vi "test_read-nmea-data2.vi"() -> ()   [LabVIEW 2019] (continued)
$GNGLL,3723.59722,N,12656.90157,E,060937.00,A,A*7E\n\t\n15:09:35.73\tF9P\t\t\n15:09:35.75\tF9P\t\t\n15:09:35.77\tF9P\t\t\n15:09:35.79\tF9P\t\t\n15:09:35.81\tF9P\t\t\n15:09:35.83\tF9P\t\t\n15:09:35.85\tF9P\t\t\n15:09:35.87\tF9P\t\t\n15:09:35.89\tF9P\t\t\n15:09:35.91\tF9P\t\t\n15:09:35.93\tF9P\t\t\n15:09:35.95\tF9P\t\t\n15:09:35.97\tF9P\t\t\n15:09:35.99\tF9P\t\t\n15:09:36.01\tF9P\t\t\n15:09:36.03\tF9P\t\t\n15:09:36.05\tF9P\t\t\n15:09:36.07\tF9P\t\t\n15:09:36.09\tF9P\t\t\n15:09:36.11\tF9P\t\t\n15:09:36.13\tF9P\t\t\n15:09:36.15\tF9P\t\t\n15:09:36.17\tF9P\t\t\n15:09:36.19\tF9P\t\t\n15:09:36.21\tF9P\t\t\n15:09:36.23\tF9P\t\t\n15:09:36.25\tF9P\t$GNRMC,060938.00,A,3723.59553,N,12656.90183,E,2.222,230.38,250720,,,A,V*09\n\t\n15:09:36.27\tF9P\t$GNVTG,230.38,T,,M,2.222,N,4.116,K,A*2B\n\t\n15:09:36.29\tF9P\t$GNGGA,060938.00,3723.59553,N,12656.90183,E,1,12,0.71,43.4,M,18.5,M,,*73\n\t\n15:09:36.31\tF9P\t$GNGSA,A,3,12,06,19,05,17,09,04,02,,,,,1.43,0.71,1.24,1*07\n\t\n15:09:36.33\tF9P\t$GNGSA,A,3,85,71,84,,,,,,,,,,1.43,0.71,1.24,2*02\n\t\n15:09:36.35\tF9P\t$GNGSA,A,3,36,19,11,04,09,12,,,,,,,1.43,0.71,1.24,3*07\n\t\n15:09:36.37\tF9P\t$GNGSA,A,3,14,11,33,,,,,,,,,,1.43,0.71,1.24,4*06\n\t\n15:09:36.39\tF9P\t$GPGSV,3,1,09,02,54,318,27,04,19,044,16,05,36,246,27,06,65,046,28,1*60\n\t\n15:09:36.41\tF9P\t$GPGSV,3,2,09,09,45,075,29,12,24,278,20,17,34,153,39,19,53,156,35,1*61\n\t\n15:09:36.43\tF9P\t$GPGSV,3,3,09,25,12,307,20,1*5F\n\t\n15:09:36.45\tF9P\t$GPGSV,3,1,09,02,54,318,,04,19,044,,05,36,246,23,06,65,046,25,6*6C\n\t\n15:09:36.47\tF9P\t$GPGSV,3,2,09,09,45,075,23,12,24,278,,17,34,153,26,19,53,156,,6*66\n\t\n15:09:36.49\tF9P\t$GPGSV,3,3,09,25,12,307,,6*5A\n\t\n15:09:36.51\tF9P\t$GLGSV,2,1,08,69,13,031,,70,73,042,,71,50,204,29,72,03,209,,1*7A\n\t\n15:09:36.53\tF9P\t$GLGSV,2,2,08,77,01,327,,84,21,121,07,85,70,063,32,86,35,329,,1*73\n\t\n15:09:36.55\tF9P\t$GLGSV,2,1,08,69,13,031,,70,73,042,,71,50,204,22,72,03,209,,3*73\n\t\n15:09:36.57\tF9P\t$GLGSV,2,2,08,77,01,327,,84,21,121,15,85,70,063,22,86,35,329,,3*73\n\t\n15:09:36.59\tF9P\t$GAGSV,2,1,08,02,09,298,15,04,66,119,33,09,30,193,22,11,70,356,24,7*79\n\t\n15:09:36.61\tF9P\t$GAGSV,2,2,08,12,41,101,19,19,27,046,13,25,10,250,,36,25,307,29,7*74\n\t\n15:09:36.63\tF9P\t$GAGSV,2,1,08,02,09,298,,04,66,119,31,09,30,193,23,11,70,356,18,2*74\n\t\n15:09:36.65\tF9P\t$GAGSV,2,2,08,12,41,101,,19,27,046,,25,10,250,,36,25,307,30,2*73\n\t\n15:09:36.67\tF9P\t$GBGSV,1,1,03,11,51,130,22,14,86,148,28,33,59,218,30,1*4B\n\t\n15:09:36.69\tF9P\t$GBGSV,1,1,04,08,,,21,11,51,130,23,14,86,148,24,33,59,218,,3*4B\n\t\n15:09:36.71\tF9P\t$GNGLL,3723.59553,N,12656.90183,E,060938.00,A,A*7C\n\t\n15:09:36.73\tF9P\t\t\n15:09:36.75\tF9P\t\t\n15:09:36.77\tF9P\t\t\n15:09:36.79\tF9P\t\t\n15:09:36.81\tF9P\t\t\n15:09:36.83\tF9P\t\t\n15:09:36.85\tF9P\t\t\n15:09:36.87\tF9P\t\t\n15:09:36.89\tF9P\t\t\n15:09:36.91\tF9P\t\t\n15:09:36.93\tF9P\t\t\n15:09:36.95\tF9P\t\t\n15:09:36.97\tF9P\t\t\n15:09:36.99\tF9P\t\t\n15:09:37.01\tF9P\t\t\n15:09:37.03\tF9P\t\t\n15:09:37.05\tF9P\t\t\n15:09:37.07\tF9P\t\t\n15:09:37.09\tF9P\t\t\n15:09:37.11\tF9P\t\t\n15:09:37.13\tF9P\t\t\n15:09:37.16\tF9P\t\t\n15:09:37.17\tF9P\t\t\n15:09:37.19\tF9P\t\t\n15:09:37.21\tF9P\t\t\n15:09:37.23\tF9P\t\t\n15:09:37.25\tF9P\t$GNRMC,060939.00,A,3723.59412,N,12656.90203,E,2.452,229.18,250720,,,A,V*0C\n\t\n15:09:37.27\tF9P\t$GNVTG,229.18,T,,M,2.452,N,4.542,K,A*25\n\t\n15:09:37.29\tF9P\t$GNGGA,060939.00,3723.59412,N,12656.90203,E,1,12,0.68,41.2,M,18.5,M,,*71\n\t\n15:09:37.31\tF9P\t$GNGSA,A,3,12,06,19,05,17,09,04,02,,,,,1.28,0.68,1.09,1*0D\n\t\n15:09:37.33\tF9P\t$GNGSA,A,3,85,71,84,,,,,,,,,,1.28,0.68,1.09,2*08\n\t\n15:09:37.35\tF9P\t$GNGSA,A,3,36,19,11,04,09,12,,,,,,,1.28,0.68,1.09,3*0D\n\t\n15:09:37.37\tF9P\t$GNGSA,A,3,14,11,33,,,,,,,,,,1.28,0.68,1.09,4*0C\n\t\n15:09:37.39\tF9P\t$GPGSV,3,1,09,02,54,318,33,04,19,044,18,05,36,246,26,06,65,046,29,1*6B\n\t\n15:09:37.41\tF9P\t$GPGSV,3,2,09,09,45,075,30,12,24,278,19,17,34,153,42,19,53,156,30,1*6A\n\t\n15:09:37.43\tF9P\t$GPGSV,3,3,09,25,12,307,19,1*55\n\t\n15:09:37.45\tF9P\t$GPGSV,3,1,09,02,54,318,,04,19,044,,05,36,246,22,06,65,046,26,6*6E\n\t\n15:09:37.47\tF9P\t$GPGSV,3,2,09,09,45,075,22,12,24,278,,17,34,153,26,19,53,156,,6*67\n\t\n15:09:37.49\tF9P\t$GPGSV,3,3,09,25,12,307,,6*5A\n\t\n15:09:37.51\tF9P\t$GLGSV,2,1,08,69,13,031,,70,73,042,,71,50,204,28,72,03,209,,1*7B\n\t\n15:09:37.53\tF9P\t$GLGSV,2,2,08,77,01,327,,84,21,121,08,85,70,063,25,86,35,329,,1*7A\n\t\n15:09:37.55\tF9P\t$GLGSV,2,1,08,69,13,031,20,70,73,042,,71,50,204,21,72,03,209,,3*72\n\t\n15:09:37.57\tF9P\t$GLGSV,2,2,08,77,01,327,,84,21,121,13,85,70,063,24,86,35,329,,3*73\n\t\n15:09:37.59\tF9P\t$GAGSV,2,1,08,02,09,298,13,04,66,119,42,09,31,193,23,11,70,356,24,7*79\n\t\n15:09:37.61\tF9P\t$GAGSV,2,2,08,12,41,101,17,19,27,046,18,25,10,250,,36,25,307,27,7*7F\n\t\n15:09:37.63\tF9P\t$GAGSV,2,1,08,02,09,298,,04,66,119,25,09,31,193,23,11,70,356,17,2*7F\n\t\n15:09:37.65\tF9P\t$GAGSV,2,2,08,12,41,101,,19,27,046,,25,10,250,,36,25,307,26,2*74\n\t\n15:09:37.67\tF9P\t$GBGSV,1,1,03,11,51,130,23,14,86,148,27,33,59,218,30,1*45\n\t\n15:09:37.69\tF9P\t$GBGSV,1,1,04,08,,,20,11,51,130,22,14,86,148,24,33,59,218,,3*4B\n\t\n15:09:37.71\tF9P\t$GNGLL,3723.59412,N,12656.90203,E,060939.00,A,A*72\n\t\n15:09:37.73\tF9P\t\t\n15:09:37.75\tF9P\t\t\n15:09:37.77\tF9P\t\t\n15:09:37.79\tF9P\t\t\n15:09:37.81\tF9P\t\t\n15:09:37.83\tF9P\t\t\n15:09:37.85\tF9P\t\t\n15:09:37.87\tF9P\t\t\n15:09:37.89\tF9P\t\t\n15:09:37.91\tF9P\t\t\n15:09:37.93\tF9P\t\t\n15:09:37.95\tF9P\t\t\n15:09:37.97\tF9P\t\t\n15:09:37.99\tF9P\t\t\n15:09:38.01\tF9P\t\t\n15:09:38.03\tF9P\t\t\n15:09:38.05\tF9P\t\t\n15:09:38.07\tF9P\t\t\n15:09:38.09\tF9P\t\t\n15:09:38.11\tF9P\t\t\n15:09:38.13\tF9P\t\t\n15:09:38.16\tF9P\t\t\n15:09:38.18\tF9P\t\t\n15:09:38.20\tF9P\t\t\n15:09:38.22\tF9P\t\t\n15:09:38.24\tF9P\t\t\n15:09:38.26\tF9P\t$GNRMC,060940.00,A,3723.59268,N,12656.90207,E,1.545,230.13,250720,,,A,V*0A\n\t\n15:09:38.28\tF9P\t$GNVTG,230.13,T,,M,1.545,N,2.862,K,A*2B\n\t\n15:09:38.30\tF9P\t$GNGGA,060940.00,3723.59268,N,12656.90207,E,1,12,0.71,39.9,M,18.5,M,,*7C\n\t\n15:09:38.32\tF9P\t$GNGSA,A,3,12,06,19,05,17,09,04,02,,,,,1.43,0.71,1.24,1*07\n\t\n15:09:38.34\tF9P\t$GNGSA,A,3,85,71,84,,,,,,,,,,1.43,0.71,1.24,2*02\n\t\n15:09:38.36\tF9P\t$GNGSA,A,3,36,19,11,04,09,12,,,,,,,1.43,0.71,1.24,3*07\n\t\n15:09:38.38\tF9P\t$GNGSA,A,3,14,11,33,,,,,,,,,,1.43,0.71,1.24,4*06\n\t\n15:09:38.40\tF9P\t$GPGSV,3,1,09,02,54,318,28,04,19,044,21,05,36,246,26,06,65,046,35,1*66\n\t\n15:09:38.42\tF9P\t$GPGSV,3,2,09,09,45,075,31,12,24,278,20,17,34,153,45,19,53,156,43,1*62\n\t\n15:09:38.44\tF9P\t$GPGSV,3,3,09,25,12,307,19,1*55\n\t\n15:09:38.46\tF9P\t$GPGSV,3,1,09,02,54,318,,04,19,044,,05,36,246,22,06,65,046,26,6*6E\n\t\n15:09:38.48\tF9P\t$GPGSV,3,2,09,09,45,075,21,12,24,278,,17,34,153,26,19,53,156,,6*64\n\t\n15:09:38.50\tF9P\t$GPGSV,3,3,09,25,12,307,,6*5A\n\t\n15:09:38.52\tF9P\t$GLGSV,2,1,08,69,13,031,,70,73,042,,71,50,204,23,72,03,209,,1*70\n\t\n15:09:38.54\tF9P\t$GLGSV,2,2,08,77,01,327,,84,21,121,07,85,70,063,31,86,35,329,,1*70\n\t\n15:09:38.56\tF9P\t$GLGSV,2,1,08,69,13,031,18,70,73,042,,71,50,204,19,72,03,209,,3*72\n\t\n15:09:38.58\tF9P\t$GLGSV,2,2,08,77,01,327,,84,21,121,16,85,70,063,25,86,35,329,,3*77\n\t\n15:09:38.60\tF9P\t$GAGSV,2,1,08,02,09,298,12,04,66,119,37,09,31,193,23,11,71,357,27,7*79\n\t\n15:09:38.62\tF9P\t$GAGSV,2,2,08,12,41,101,25,19,27,046,10,25,10,250,,36,25,307,26,7*77\n\t\n15:09:38.64\tF9P\t$GAGSV,2,1,08,02,09,298,,04,66,119,25,09,31,193,21,11,71,357,16,2*7C\n\t\n15:09:38.66\tF9P\t$GAGSV,2,2,08,12,41,101,,19,27,046,,25,10,250,,36,25,307,25,2*77\n\t\n15:09:38.68\tF9P\t$GBGSV,1,1,03,11,51,130,21,14,86,148,28,33,59,218,29,1*40\n\t\n15:09:38.70\tF9P\t$GBGSV,1,1,04,08,,,19,11,51,130,20,14,86,148,22,33,59,218,,3*45\n\t\n15:09:38.72\tF9P\t$GNGLL,3723.59268,N,12656.90207,E,060940.00,A,A*73\n\t\n15:09:38.74\tF9P\t\t\n15:09:38.76\tF9P\t\t\n15:09:38.78\tF9P\t\t\n15:09:38.80\tF9P\t\t\n15:09:38.82\tF9P\t\t\n15:09:38.84\tF9P\t\t\n15:09:38.86\tF9P\t\t\n15:09:38.88\tF9P\t\t\n15:09:38.90\tF9P\t\t\n15:09:38.92\tF9P\t\t\n15:09:38.94\tF9P\t\t\n15:09:38.96\tF9P\t\t\n15:09:38.98\tF9P\t\t\n15:09:39.00\tF9P\t\t\n15:09:39.02\tF9P\t\t\n15:09:39.04\tF9P\t\t\n15:09:39.06\tF9P\t\t\n15:09:39.08\tF9P\t\t\n15:09:39.10\tF9P\t\t\n15:09:39.12\tF9P\t\t\n15:09:39.14\tF9P\t\t\n15:09:39.16\tF9P\t\t\n15:09:39.18\tF9P\t\t\n15:09:39.20\tF9P\t\t\n15:09:39.22\tF9P\t\t\n15:09:39.24\tF9P\t\t\n15:09:39.26\tF9P\t$GNRMC,060941.00,A,3723.59186,N,12656.90135,E,1.647,232.79,250720,,,A,V*05\n\t\n15:09:39.28\tF9P\t$GNVTG,232.79,T,,M,1.647,N,3.050,K,A*2C\n\t\n15:09:39.30\tF9P\t$GNGGA,060941.00,3723.59186,N,12656.90135,E,1,12,0.72,41.6,M,18.5,M,,*7F\n\t\n15:09:39.32\tF9P\t$GNGSA,A,3,12,06,19,05,17,09,04,02,,,,,1.36,0.72,1.16,1*07\n\t\n15:09:39.34\tF9P\t$GNGSA,A,3,85,71,84,,,,,,,,,,1.36,0.72,1.16,2*02\n\t\n15:09:39.36\tF9P\t$GNGSA,A,3,36,19,11,04,09,12,,,,,,,1.36,0.72,1.16,3*07\n\t\n15:09:39.38\tF9P\t$GNGSA,A,3,14,11,33,,,,,,,,,,1.36,0.72,1.16,4*06\n\t\n15:09:39.40\tF9P\t$GPGSV,3,1,09,02,54,318,28,04,19,044,24,05,36,246,27,06,65,046,33,1*64\n\t\n15:09:39.42\tF9P\t$GPGSV,3,2,09,09,45,075,35,12,24,278,22,17,34,153,30,19,53,156,39,1*6B\n\t\n15:09:39.44\tF9P\t$GPGSV,3,3,09,25,12,307,19,1*55\n\t\n15:09:39.46\tF9P\t$GPGSV,3,1,09,02,54,318,,04,19,044,,05,36,246,24,06,65,046,28,6*66\n\t\n15:09:39.48\tF9P\t$GPGSV,3,2,09,09,45,075,23,12,24,278,,17,34,153,25,19,53,156,,6*65\n\t\n15:09:39.50\tF9P\t$GPGSV,3,3,09,25,12,307,,6*5A\n\t\n15:09:39.52\tF9P\t$GLGSV,2,1,08,69,13,031,,70,73,042,,71,50,204,25,72,03,209,,1*76\n\t\n15:09:39.54\tF9P\t$GLGSV,2,2,08,77,01,327,,84,21,121,10,85,70,063,25,86,35,329,,1*73\n\t\n15:09:39.56\tF9P\t$GLGSV,2,1,08,69,13,031,17,70,73,042,,71,50,204,18,72,03,209,,3*7C\n\t\n15:09:39.58\tF9P\t$GLGSV,2,2,08,77,01,327,,84,21,121,16,85,70,063,23,86,35,329,,3*71\n\t\n15:09:39.60\tF9P\t$GAGSV,2,1,08,02,09,298,14,04,66,119,29,09,31,193,24,11,71,357,20,7*70\n\t\n15:09:39.62\tF9P\t$GAGSV,2,2,08,12,40,102,19,19,27,046,19,25,10,250,,36,25,307,26,7*73\n\t\n15:09:39.64\tF9P\t$GAGSV,2,1,08,02,09,298,,04,66,119,,09,31,193,21,11,71,357,16,2*7B\n\t\n15:09:39.66\tF9P\t$GAGSV,2,2,08,12,40,102,,19,27,046,,25,10,250,,36,25,307,25,2*75\n\t\n15:09:39.68\tF9P\t$GBGSV,1,1,03,11,51,130,22,14,86,148,33,33,59,218,27,1*47\n\t\n15:09:39.70\tF9P\t$GBGSV,1,1,04,08,,,21,11,51,130,21,14,86,148,23,33,59,218,,3*4E\n\t\n15:09:39.72\tF9P\t$GNGLL,3723.59186,N,12656.90135,E,060941.00,A,A*73\n\t\n15:09:39.74\tF9P\t\t\n15:09:39.76\tF9P\t\t\n15:09:39.78\tF9P\t\t\n15:09:39.80\tF9P\t\t\n15:09:39.82\tF9P\t\t\n15:09:39.84\tF9P\t\t\n15:09:39.86\tF9P\t\t\n15:09:39.88\tF9P\t\t\n15:09:39.90\tF9P\t\t\n15:09:39.92\tF9P\t\t\n15:09:39.94\tF9P\t\t\n15:09:39.96\tF9P\t\t\n15:09:39.98\tF9P\t\t\n15:09:40.00\tF9P\t\t\n15:09:40.02\tF9P\t\t\n15:09:40.04\tF9P\t\t\n15:09:40.06\tF9P\t\t\n15:09:40.08\tF9P\t\t\n15:09:40.10\tF9P\t\t\n15:09:40.12\tF9P\t\t\n15:09:40.14\tF9P\t\t\n15:09:40.16\tF9P\t\t\n15:09:40.18\tF9P\t\t\n15:09:40.20\tF9P\t\t\n15:09:40.22\tF9P\t\t\n15:09:40.24\tF9P\t\t\n15:09:40.26\tF9P\t$GNRMC,060942.00,A,3723.59138,N,12656.90085,E,1.607,230.05,250720,,,A,V*04\n\t\n15:09:40.28\tF9P\t$GNVTG,230.05,T,,M,1.607,N,2.977,K,A*2C\n\t\n15:09:40.30\tF9P\t$GNGGA,060942.00,3723.59138,N,12656.90085,E,1,12,0.72,42.4,M,18.5,M,,*72\n\t\n15:09:40.32\tF9P\t$GNGSA,A,3,12,06,19,05,17,09,04,02,,,,,1.36,0.72,1.16,1*07\n\t\n15:09:40.34\tF9P\t$GNGSA,A,3,85,71,84,,,,,,,,,,1.36,0.72,1.16,2*02\n\t\n15:09:40.36\tF9P\t$GNGSA,A,3,36,19,11,04,09,12,,,,,,,1.36,0.72,1.16,3*07\n\t\n15:09:40.38\tF9P\t$GNGSA,A,3,14,11,33,,,,,,,,,,1.36,0.72,1.16,4*06\n\t\n15:09:40.40\tF9P\t$GPGSV,3,1,09,02,54,318,32,04,19,044,22,05,36,246,25,06,65,046,35,1*6D\n\t\n15:09:40.42\tF9P\t$GPGSV,3,2,09,09,45,075,31,12,24,278,21,17,34,153,30,19,53,156,31,1*64\n\t\n15:09:40.44\tF9P\t$GPGSV,3,3,09,25,12,307,20,1*5F\n\t\n15:09:40.46\tF9P\t$GPGSV,3,1,09,02,54,318,,04,19,044,23,05,36,246,26,06,65,046,26,6*6B\n\t\n15:09:40.48\tF9P\t$GPGSV,3,2,09,09,45,075,22,12,24,278,,17,34,153,,19,53,156,,6*63\n\t\n15:09:40.50\tF9P\t$GPGSV,3,3,09,25,12,307,,6*5A\n\t\n15:09:40.52\tF9P\t$GLGSV,2,1,08,69,13,031,,70,73,042,,71,50,204,35,72,03,209,,1*77\n\t\n15:09:40.54\tF9P\t$GLGSV,2,2,08,77,01,327,,84,21,121,10,85,70,063,26,86,35,329,,1*70\n\t\n15:09:40.56\tF9P\t$GLGSV,2,1,08,69,13,031,18,70,73,042,,71,50,204,17,72,03,209,,3*7C\n\t\n15:09:40.58\tF9P\t$GLGSV,2,2,08,77,01,327,,84,21,121,16,85,70,063,23,86,35,329,,3*71\n\t\n15:09:40.60\tF9P\t$GAGSV,2,1,08,02,09,298,15,04,66,119,34,09,31,193,24,11,71,357,20,7*7D\n\t\n15:09:40.62\tF9P\t$GAGSV,2,2,08,12,40,102,18,19,27,046,19,25,10,250,,36,25,307,27,7*73\n\t\n15:09:40.64\tF9P\t$GAGSV,2,1,08,02,09,298,,04,66,119,,09,31,193,18,11,71,357,16,2*71\n\t\n15:09:40.66\tF9P\t$GAGSV,2,2,08,12,40,102,,19,27,046,,25,10,250,,36,25,307,22,2*72\n\t\n15:09:40.68\tF9P\t$GBGSV,1,1,03,11,51,130,26,14,86,148,27,33,59,218,32,1*42\n\t\n15:09:40.70\tF9P\t$GBGSV,1,1,04,08,,,21,11,51,130,21,14,86,148,22,33,59,218,,3*4F\n\t\n15:09:40.72\tF9P\t$GNGLL,3723.59138,N,12656.90085,E,060942.00,A,A*7F\n\t\n15:09:40.74\tF9P\t\t\n15:09:40.76\tF9P\t\t\n15:09:40.78\tF9P\t\t\n15:09:40.80\tF9P\t\t\n15:09:40.82\tF9P\t\t\n15:09:40.84\tF9P\t\t\n15:09:40.86\tF9P\t\t\n15:09:40.88\tF9P\t\t\n15:09:40.90\tF9P\t\t\n15:09:40.92\tF9P\t\t\n15:09:40.94\tF9P\t\t\n15:09:40.96\tF9P\t\t\n15:09:40.98\tF9P\t\t\n15:09:41.00\tF9P\t\t\n15:09:41.02\tF9P\t\t\n15:09:41.04\tF9P\t\t\n15:09:41.06\tF9P\t\t\n15:09:41.08\tF9P\t\t\n15:09:41.10\tF9P\t\t\n15:09:41.12\tF9P\t\t\n15:09:41.14\tF9P\t\t\n15:09:41.16\tF9P\t\t\n15:09:41.18\tF9P\t\t\n15:09:41.20\tF9P\t\t\n15:09:41.22\tF9P\t\t\n15:09:41.24\tF9P\t\t\n15:09:41.26\tF9P\t$GNRMC,060943.00,A,3723.59098,N,12656.90017,E,2.065,236.92,250720,,,A,V*0C\n\t\n15:09:41.28\tF9P\t$GNVTG,236.92,T,,M,2.065,N,3.824,K,A*23\n\t\n15:09:41.30\tF9P\t$GNGGA,060943.00,3723.59098,N,12656.90017,E,1,12,0.75,42.8,M,18.5,M,,*78\n\t\n15:09:41.32\tF9P\t$GNGSA,A,3,12,06,19,05,17,09,04,02,,,,,1.51,0.75,1.31,1*04\n\t\n15:09:41.34\tF9P\t$GNGSA,A,3,85,71,84,,,,,,,,,,1.51,0.75,1.31,2*01\n\t\n15:09:41.36\tF9P\t$GNGSA,A,3,36,19,11,04,09,12,,,,,,,1.51,0.75,1.31,3*04\n\t\n15:09:41.38\tF9P\t$GNGSA,A,3,14,11,33,,,,,,,,,,1.51,0.75,1.31,4*05\n\t\n15:09:41.40\tF9P\t$GPGSV,3,1,09,02,54,318,30,04,19,044,21,05,36,246,25,06,65,046,31,1*68\n\t\n15:09:41.42\tF9P\t$GPGSV,3,2,09,09,45,075,31,12,24,278,21,17,34,153,29,19,53,156,34,1*69\n\t\n15:09:41.44\tF9P\t$GPGSV,3,3,09,25,12,307,21,1*5E\n\t\n15:09:41.46\tF9P\t$GPGSV,3,1,09,02,54,318,,04,19,044,19,05,36,246,27,06,65,046,26,6*63\n\t\n15:09:41.48\tF9P\t$GPGSV,3,2,09,09,45,075,22,12,24,278,,17,34,153,,19,53,156,,6*63\n\t\n15:09:41.50\tF9P\t$GPGSV,3,3,09,25,12,307,,6*5A\n\t\n15:09:41.52\tF9P\t$GLGSV,2,1,08,69,13,031,,70,73,042,,71,50,204,26,72,03,209,,1*75\n\t\n15:09:41.54\tF9P\t$GLGSV,2,2,08,77,01,327,,84,21,121,11,85,70,063,26,86,35,329,,1*71\n\t\n15:09:41.56\tF9P\t$GLGSV,2,1,08,69,13,031,16,70,73,042,,71,50,204,19,72,03,209,,3*7C\n\t\n15:09:41.58\tF9P\t$GLGSV,2,2,08,77,01,327,,84,21,121,17,85,70,063,23,86,35,329,,3*70\n\t\n15:09:41.60\tF9P\t$GAGSV,2,1,08,02,09,298,15,04,66,119,33,09,31,193,24,11,71,357,22,7*78\n\t\n15:09:41.62\tF9P\t$GAGSV,2,2,08,12,40,102,19,19,27,046,18,25,10,250,,36,25,307,25,7*71\n\t\n15:09:41.64\tF9P\t$GAGSV,2,1,08,02,09,298,,04,66,119,,09,31,193,18,11,71,357,16,2*71\n\t\n15:09:41.66\tF9P\t$GAGSV,2,2,08,12,40,102,,19,27,046,,25,10,250,,36,25,307,24,2*74\n\t\n15:09:41.68\tF9P\t$GBGSV,1,1,03,11,51,130,25,14,86,148,25,33,59,218,32,1*43\n\t\n15:09:41.70\tF9P\t$GBGSV,1,1,04,08,,,20,11,51,130,21,14,86,148,28,33,59,218,,3*44\n\t\n15:09:41.72\tF9P\t$GNGLL,3723.59098,N,12656.90017,E,060943.00,A,A*7E\n\t\n15:09:41.74\tF9P\t\t\n15:09:41.76\tF9P\t\t\n15:09:41.78\tF9P\t\t\n15:09:41.80\tF9P\t\t\n15:09:41.82\tF9P\t\t\n15:09:41.84\tF9P\t\t\n15:09:41.86\tF9P\t\t\n15:09:41.88\tF9P\t\t\n15:09:41.90\tF9P\t\t\n15:09:41.92\tF9P\t\t\n15:09:41.94\tF9P\t\t\n15:09:41.96\tF9P\t\t\n15:09:41.98\tF9P\t\t\n15:09:42.00\tF9P\t\t\n15:09:42.02\tF9P\t\t\n15:09:42.04\tF9P\t\t\n15:09:42.06\tF9P\t\t\n15:09:42.08\tF9P\t\t\n15:09:42.10\tF9P\t\t\n15:09:42.12\tF9P\t\t\n15:09:42.14\tF9P\t\t\n15:09:42.16\tF9P\t\t\n15:09:42.18\tF9P\t\t\n15:09:42.20\tF9P\t\t\n15:09:42.22\tF9P\t\t\n15:09:42.24\tF9P\t\t\n15:09:42.26\tF9P\t$GNRMC,060944.00,A,3723.59080,N,12656.89955,E,1.383,241.70,250720,,,A,V*01\n\t\n15:09:42.28\tF9P\t$GNVTG,241.70,T,,M,1.383,N,2.562,K,A*29\n\t\n15:09:42.30\tF9P\t$GNGGA,060944.00,3723.59080,N,12656.89955,E,1,12,0.74,42.6,M,18.5,M,,*7E\n\t\n15:09:42.32\tF9P\t$GNGSA,A,3,12,06,19,05,17,09,02,,,,,,1.39,0.74,1.18,1*04\n\t\n15:09:42.34\tF9P\t$GNGSA,A,3,85,71,84,,,,,,,,,,1.39,0.74,1.18,2*05\n\t\n15:09:42.36\tF9P\t$GNGSA,A,3,36,19,11,04,09,12,,,,,,,1.39,0.74,1.18,3*00\n\t\n15:09:42.38\tF9P\t$GNGSA,A,3,14,11,33,,,,,,,,,,1.39,0.74,1.18,4*01\n\t\n15:09:42.40\tF9P\t$GPGSV,3,1,09,02,54,318,23,04,19,044,21,05,36,246,23,06,65,046,27,1*6B\n\t\n15:09:42.42\tF9P\t$GPGSV,3,2,09,09,45,075,31,12,24,278,22,17,34,153,34,19,53,156,36,1*64\n\t\n15:09:42.44\tF9P\t$GPGSV,3,3,09,25,12,307,20,1*5F\n\t\n15:09:42.46\tF9P\t$GPGSV,3,1,09,02,54,318,,04,19,044,16,05,36,246,32,06,65,046,26,6*68\n\t\n15:09:42.48\tF9P\t$GPGSV,3,2,09,09,45,075,24,12,24,278,,17,34,153,21,19,53,156,,6*66\n\t\n15:09:42.50\tF9P\t$GPGSV,3,3,09,25,12,307,,6*5A\n\t\n15:09:42.52\tF9P\t$GLGSV,2,1,08,69,13,031,,70,73,042,,71,50,204,27,72,03,209,,1*74\n\t\n15:09:42.54\tF9P\t$GLGSV,2,2,08,77,01,327,,84,21,121,11,85,70,063,24,86,35,329,,1*73\n\t\n15:09:42.56\tF9P\t$GLGSV,2,1,08,69,13,031,13,70,73,042,,71,50,204,20,72,03,209,,3*73\n\t\n15:09:42.58\tF9P\t$GLGSV,2,2,08,77,01,327,,84,21,121,18,85,70,063,21,86,35,329,,3*7D\n\t\n15:09:42.60\tF9P\t$GAGSV,2,1,08,02,09,298,15,04,66,119,30,09,31,193,23,11,71,357,23,7*7D\n\t\n15:09:42.62\tF9P\t$GAGSV,2,2,08,12,40,102,19,19,27,045,15,25,10,250,,36,25,307,24,7*7E\n\t\n15:09:42.64\tF9P\t$GAGSV,2,1,08,02,09,298,,04,66,119,,09,31,193,17,11,71,357,18,2*70\n\t\n15:09:42.66\tF9P\t$GAGSV,2,2,08,12,40,102,,19,27,045,,25,10,250,,36,25,307,23,2*70\n\t\n15:09:42.68\tF9P\t$GBGSV,1,1,03,11,51,130,27,14,86,148,30,33,59,218,27,1*41\n\t\n15:09:42.70\tF9P\t$GBGSV,1,1,04,08,,,20,11,51,130,23,14,86,148,27,33,59,218,,3*49\n\t\n15:09:42.72\tF9P\t$GNGLL,3723.59080,N,12656.89955,E,060944.00,A,A*77\n\t\n15:09:42.74\tF9P\t\t\n15:09:42.76\tF9P\t\t\n15:09:42.78\tF9P\t\t\n15:09:42.80\tF9P\t\t\n15:09:42.82\tF9P\t\t\n15:09:42.84\tF9P\t\t\n15:09:42.86\tF9P\t\t\n15:09:42.88\tF9P\t\t\n15:09:42.90\tF9P\t\t\n15:09:42.92\tF9P\t\t\n15:09:42.94\tF9P\t\t\n15:09:42.96\tF9P\t\t\n15:09:42.98\tF9P\t\t\n15:09:43.00\tF9P\t\t\n15:09:43.02\tF9P\t\t\n15:09:43.04\tF9P\t\t\n15:09:43.06\tF9P\t\t\n15:09:43.08\tF9P\t\t\n15:09:43.10\tF9P\t\t\n15:09:43.12\tF9P\t\t\n15:09:43.14\tF9P\t\t\n15:09:43.16\tF9P\t\t\n15:09:43.18\tF9P\t\t\n15:09:43.20\tF9P\t\t\n15:09:43.22\tF9P\t\t\n15:09:43.24\tF9P\t\t\n15:09:43.26\tF9P\t$GNRMC,060945.00,A,3723.59050,N,12656.89866,E,2.219,243.56,250720,,,A,V*0B\n\t\n15:09:43.28\tF9P\t$GNVTG,243.56,T,,M,2.219,N,4.109,K,A*21\n\t\n15:09:43.30\tF9P\t$GNGGA,060945.00,3723.59050,N,12656.89866,E,1,12,0.75,42.3,M,18.5,M,,*77\n\t\n15:09:43.32\tF9P\t$GNGSA,A,3,12,06,19,05,17,09,04,02,,,,,1.51,0.75,1.31,1*04\n\t\n15:09:43.34\tF9P\t$GNGSA,A,3,85,71,84,,,,,,,,,,1.51,0.75,1.31,2*01\n\t\n15:09:43.36\tF9P\t$GNGSA,A,3,36,19,11,04,09,12,,,,,,,1.51,0.75,1.31,3*04\n\t\n15:09:43.38\tF9P\t$GNGSA,A,3,14,11,33,,,,,,,,,,1.51,0.75,1.31,4*05\n\t\n15:09:43.40\tF9P\t$GPGSV,3,1,09,02,54,318,30,04,19,044,22,05,36,246,31,06,65,046,32,1*6D\n\t\n15:09:43.42\tF9P\t$GPGSV,3,2,09,09,45,075,27,12,24,278,21,17,34,153,24,19,53,156,39,1*6E\n\t\n15:09:43.44\tF9P\t$GPGSV,3,3,09,25,12,307,20,1*5F\n\t\n15:09:43.46\tF9P\t$GPGSV,3,1,09,02,54,318,,04,19,044,14,05,36,246,29,06,65,046,24,6*62\n\t\n15:09:43.48\tF9P\t$GPGSV,3,2,09,09,45,075,24,12,24,278,,17,34,153,18,19,53,156,,6*6C\n\t\n15:09:43.50\tF9P\t$GPGSV,3,3,09,25,12,307,,6*5A\n\t\n15:09:43.52\tF9P\t$GLGSV,2,1,08,69,13,031,,70,73,042,,71,50,204,26,72,03,209,,1*75\n\t\n15:09:43.54\tF9P\t$GLGSV,2,2,08,77,01,327,,84,21,121,06,85,70,063,24,86,35,329,,1*75\n\t\n15:09:43.56\tF9P\t$GLGSV,2,1,08,69,13,031,12,70,73,042,,71,50,204,21,72,03,209,,3*73\n\t\n15:09:43.58\tF9P\t$GLGSV,2,2,08,77,01,327,,84,
